vi "Create Msg Queue__ogtk.vi"(4 "error in (no error)":errorcluster, 5 "return existing (F)":bool, 6 "size (unbounded)":i32=-1, 7 "name (unnamed)":string) -> (0 "error out":errorcluster, 1 "created new":bool, 3 "msg queue":T1)   [LabVIEW 2011]
doc: "Looks up an existing message queue or creates a new message queue and returns a refnum that you can use when calling other message queue VIs."
uses:
  Msg Queue RefNum__ogtk.ctl
panel:
  # "[OpenG VI Tags] ***Do Not Remove***"
  # "Create Msg Queue.vi\n\nLooks up an existing message queue or creates a new message queue and returns a\n\nPlease visit http://www.OpenG.org to learn about the\nOpen Source LabVIEW software movement.\n\nNOTICE -- YOU MUST LEAVE THIS NOTICE IN PLACE.  PER THE TERMS OF THE LICENSE BELOW, YOU MAY SUBLICENSE THIS SOFTWARE \nIN ANY WAY THAT DOES NOT CONFLICT WITH THIS LICENSE.\n\n### BSD License (http://www.opensource.org/licenses/bsd-license.php) Begin ###\n\nCopyright (c) 2002, Jim Kring <jim@jimkring.com>\n\nAll rights reserved.\n\nRedistribution and use in source and binary forms, with or without modification, are permitted provided that the following conditions are met:\n\n    * Redistributions of source code must retain the above copyright notice, this list of conditions and the following disclaimer.\n    * Redistributions in binary form must reproduce the above copyright notice, this list of conditions and the following disclaimer in the \n       documentation and/or other materials provided with the distribution.\n    * Neither the name of SciWare, James Kring, Inc., nor the names of its contributors may be used to endorse or promote products derived \n       from this software without specific prior written permission.\n\nTHIS SOFTWARE IS PROVIDED BY THE COPYRIGHT HOLDERS AND CONTRIBUTORS \"AS IS\" AND ANY EXPRESS OR IMPLIED WARRANTIES, \nINCLUDING, BUT NOT LIMITED TO, THE IMPLIED WARRANTIES OF MERCHANTABILITY AND FITNESS FOR A PARTICULAR PURPOSE ARE \nDISCLAIMED. IN NO EVENT SHALL THE COPYRIGHT OWNER OR CONTRIBUTORS BE LIABLE FOR ANY DIRECT, INDIRECT, INCIDENTAL,\n SPECIAL, EXEMPLARY, OR CONSEQUENTIAL DAMAGES (INCLUDING, BUT NOT LIMITED TO, PROCUREMENT OF SUBSTITUTE GOODS OR \nSERVICES; LOSS OF USE, DATA, OR PROFITS; OR BUSINESS INTERRUPTION) HOWEVER CAUSED AND ON ANY THEORY OF LIABILITY, \nWHETHER IN CONTRACT, STRICT LIABILITY, OR TORT (INCLUDING NEGLIGENCE OR OTHERWISE) ARISING IN ANY WAY OUT OF THE USE \nOF THIS SOFTWARE, EVEN IF ADVISED OF THE POSSIBILITY OF SUCH DAMAGE.\n\n### BSD License End ###"
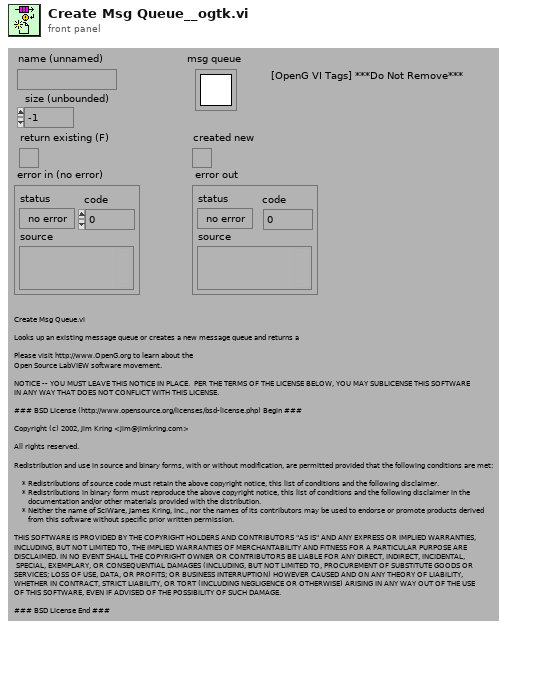
[diagram p1: front panel]
types:
  T1 = typedef "Msg Queue RefNum__ogtk.ctl" = refnum<k1>
  T2 = typedef "Queue RefNum" = refnum<k1>
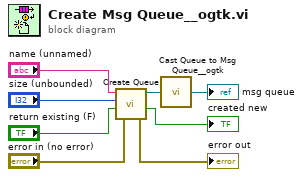
[diagram p0: block diagram]
diagram:
  n1 = call <vilib>:"Create Queue.vi"("error in (no error)"="error in (no error)", "return existing (F)"="return existing (F)", "size (unbounded)"="size (unbounded)", "name (unnamed)"="name (unnamed)") -> ("error out"=→"error out":errorcluster, "created new"=→"created new":bool, "queue out"=w2:T2)  [unwired: 1 in]
  n2 = call "Cast Queue to Msg Queue__ogtk.vi"("queue"=w2) -> ("msg queue"=→"msg queue":T1)  [unwired: 4 in]
